vi "InitionalizeInstruments3D.vi"(0 "Address 1":refnum<visa-resource-name>, 1 "Address 2":refnum<visa-resource-name>, 2 "Address 3":refnum<visa-resource-name>, 3 "Driver 1":path, 4 "Driver 2":path, 7 "error in (no error)":errorcluster, 9 "Driver 3":path) -> (20 "Instrument out":refnum<class "Instrument.lvclass">, 21 "Instrument out 2":refnum<class "Instrument.lvclass">, 22 "Instrument out 3":refnum<class "Instrument.lvclass">, 27 "error out":errorcluster)   [LabVIEW 2014]
uses:
  Classes/Abstract/Instrument/Instrument/Instrument.lvclass
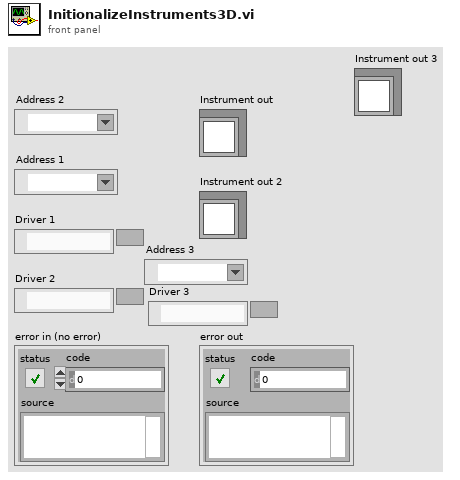
[diagram p1: front panel]
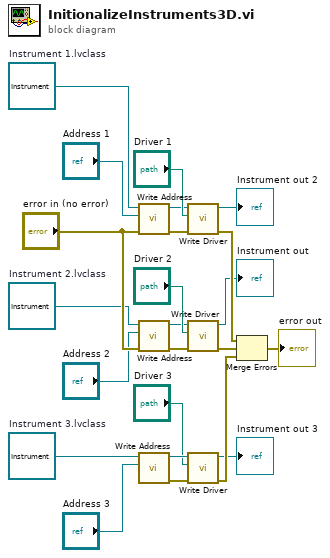
[diagram p0: block diagram]
diagram:
  w6 = refnum<class "Instrument.lvclass"> refnum  # Instrument 3.lvclass
  w10 = refnum<class "Instrument.lvclass"> refnum  # Instrument 2.lvclass
  w8 = refnum<class "Instrument.lvclass"> refnum  # Instrument 1.lvclass
  n1 = call-dynamic "Write Address.vi"("error in (no error)"="error in (no error)", "Address"="Address 1", "Instrument in"=w8) -> ("error out"=w19:errorcluster, "Instrument out"=w14:refnum<class "Instrument.lvclass">)  [unwired: 7 in]
  n2 = call-dynamic "Write Address.vi"("error in (no error)"="error in (no error)", "Address"="Address 2", "Instrument in"=w10) -> ("error out"=w18:errorcluster, "Instrument out"=w12:refnum<class "Instrument.lvclass">)  [unwired: 7 in]
  n3 = call-dynamic "Write Address.vi"("Address"="Address 3", "Instrument in"=w6) -> ("error out"=w2:errorcluster, "Instrument out"=w7:refnum<class "Instrument.lvclass">)  [unwired: 8 in]
  n4 = call-dynamic "Write Driver.vi"("error in (no error)"=w19, "Driver"="Driver 1", "Instrument in"=w14) -> ("error out"=w20:errorcluster, "Instrument out"=→"Instrument out 2":refnum<class "Instrument.lvclass">)  [unwired: 7 in]
  n5 = call-dynamic "Write Driver.vi"("error in (no error)"=w18, "Driver"="Driver 2", "Instrument in"=w12) -> ("error out"=w21:errorcluster, "Instrument out"=→"Instrument out":refnum<class "Instrument.lvclass">)  [unwired: 7 in]
  n6 = call-dynamic "Write Driver.vi"("error in (no error)"=w2, "Driver"="Driver 3", "Instrument in"=w7) -> ("error out"=w3:errorcluster, "Instrument out"=→"Instrument out 3":refnum<class "Instrument.lvclass">)  [unwired: 7 in]
  n7 = Merge Errors(w20, w21, w3) -> (→"error out":errorcluster)
